vi "Test Analog Input.vi"(8 "error in":errorcluster, 10 "TestCase in":refnum<class "Scan Engine Scripting API Modules.lvclass">, 11 "module test in":refnum<class "Module Test.lvclass">) -> (0 "error out":errorcluster, 2 "TestCase out":refnum<class "Scan Engine Scripting API Modules.lvclass">, 3 "module test out":refnum<class "Module Test.lvclass">)   [LabVIEW 2017, in "Module Test.lvclass"]
uses:
  Module Test.lvclass
  Scan Engine Scripting API Modules.lvclass
  C:/Program Files (x86)/National Instruments/LabVIEW 2017/vi.lib/addons/_JKI Toolkits/VI Tester/TestCase.llb/TestCase.lvclass
  Scripting/Modules/Mode Classes/Controls/analog channel settings.ctl
  Module Test.lvclass/Module Test.ctl
  Scripting/Scan Engine Scripting.lvlib
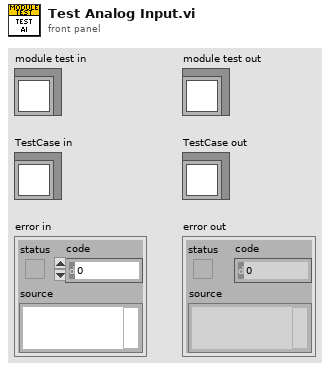
[diagram p1: front panel]
types:
  T1 = typedef "Scan Engine Scripting.lvlib/analog channel settings.ctl" = cluster{"name":string, "default value":dbl}
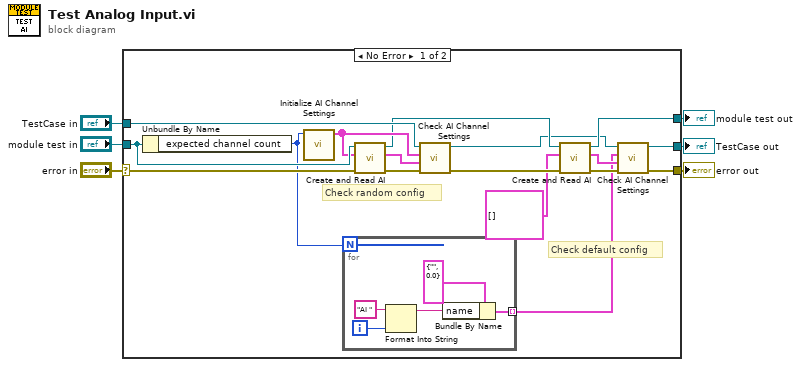
[diagram p0: block diagram]
diagram:
  n1 = case shown="No Error" "error in" {
    selector: "error in" -> [w20 w31]
    tunnel: [w14 w31] -> w5
    tunnel: [w15 w30] -> w3
    tunnel: "module test in" -> [w23 w30]
    tunnel: "TestCase in" -> [w22 w29]
    tunnel: [w11 w29] -> w1
    frame No Error {
      # "Check default config"
      # "Check random config"
      n2 = Unbundle By Name(w23) -> ("expected channel count"=w9:i32)
      n3 = call "Initialize AI Channel Settings.vi"("array size"=w9) -> ("channel settings"=w21:T1[])  [unwired: 10 in]
      n4 = for {
        N: w9 -> [_]
        tunnel: [w24] -> w8 mode=indexing
        i -> [w27]
        n5 = Format Into String(initial string="AI ", w27) -> (resulting string=w25:string)  [unwired: 2 in, 1 out]
        n6 = Bundle By Name(cluster=T1 {"name"="", "default value"=0.0} ("channel settings"), "name"=w25) -> (w24:T1)
      }
      n7 = call-dynamic "Create and Read AI.vi"("error in"=w20, "initial channel settings"=w21, "module test in"=w23) -> ("error out"=w19:errorcluster, "read channel settings"=w18:T1[], "module test out"=w17:refnum<class "Module Test.lvclass">)  [unwired: 6 in]
      n8 = call "Check AI Channel Settings.vi"("error in"=w19, "read channel settings"=w18, "initial channel settings"=w21, "TestCase in"=w22) -> ("error out"=w16:errorcluster, "TestCase out"=w12:refnum<class "Scan Engine Scripting API Modules.lvclass">)  [unwired: 6 in]
      n9 = call-dynamic "Create and Read AI.vi"("error in"=w16, "initial channel settings"=T1[] [], "module test in"=w17) -> ("error out"=w13:errorcluster, "read channel settings"=w10:T1[], "module test out"=w15:refnum<class "Module Test.lvclass">)  [unwired: 6 in]
      n10 = call "Check AI Channel Settings.vi"("error in"=w13, "read channel settings"=w10, "initial channel settings"=w8, "TestCase in"=w12) -> ("error out"=w14:errorcluster, "TestCase out"=w11:refnum<class "Scan Engine Scripting API Modules.lvclass">)  [unwired: 6 in]
    }
    frame Error {
    }
  }
  "error out" <- w5
  "module test out" <- w3
  "TestCase out" <- w1
